vi "Write connect.vi"(8 "error in (no error)":errorcluster, 10 "connect":bool, 11 "Master CR in":refnum<class "Master CR.lvclass">) -> (0 "error out":errorcluster, 3 "Master CR out":refnum<class "Master CR.lvclass">)   [LabVIEW 2021, in "Master CR.lvclass"]
uses:
  Master CR.lvclass
  Master CR.lvclass/Master CR.ctl
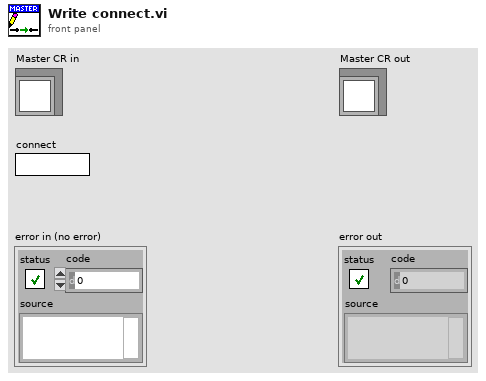
[diagram p1: front panel]
types:
  T1 = typedef "Master CR.lvclass/MB state.ctl" = cluster{"state":T2, "enable":bool, "write enable":bool, "connect":bool, "errors":i32}
  T2 = typedef "Master CR.lvclass/MB_TCP_State.ctl" = enum8{"initialization", "redefine", "standby", "ping", "connect", "wait to reconnect", "wait to reset timeout", "configure", "requests", "close connection", "stop"}
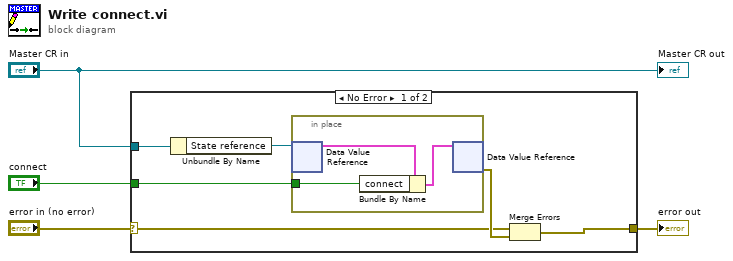
[diagram p0: block diagram]
diagram:
  n1 = case shown="No Error" "error in (no error)" {
    selector: "error in (no error)" -> [w5 w14]
    tunnel: [w8 w14] -> w3
    tunnel: "Master CR in" -> [w6 _]
    tunnel: "connect" -> [w7 _]
    frame No Error {
      n2 = Unbundle By Name(w6) -> ("State reference"=w10:refnum<data-value>)
      n3 = in-place {
        in-place-border: w7 -> [w11]
        n4 = in-place-dvr #1(w10) -> (w13:T1)  [unwired: 1 out]
        n5 = Bundle By Name(cluster=w13, "connect"=w11) -> (w12:T1)
        n6 = in-place-dvr #1(w12) -> (w9:errorcluster)  [unwired: 1 out]
      }
      n7 = Merge Errors(w5, w9) -> (w8:errorcluster)
    }
    frame Error {
    }
  }
  "error out" <- w3
  "Master CR out" <- "Master CR in"
